vi "Write VISA Resource.vi"(8 "error in (no error)":errorcluster, 10 "VISA Resource":refnum<visa-resource-name>, 11 "Instrument.lvclass in":refnum<class "Instrument.lvclass">) -> (0 "error out":errorcluster, 3 "Instrument.lvclass out":refnum<class "Instrument.lvclass">)   [LabVIEW 2015, in "Instrument.lvclass"]
uses:
  Instrument.lvclass
  Instrument.lvclass/Instrument.ctl
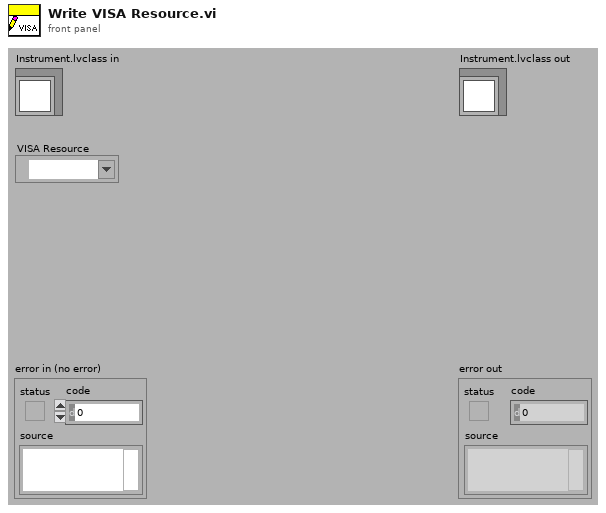
[diagram p1: front panel]
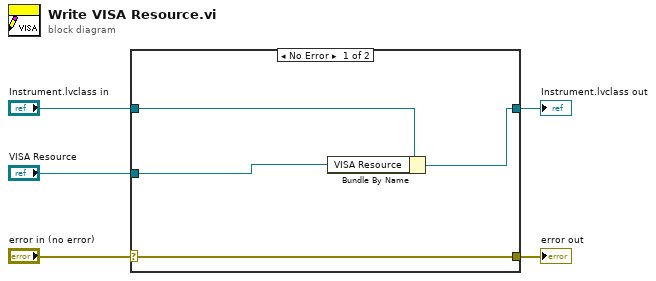
[diagram p0: block diagram]
diagram:
  n1 = case shown="No Error" "error in (no error)" {
    selector: "error in (no error)" -> [w9 w10]
    tunnel: [w9 w10] -> w4
    tunnel: [w7 w11] -> w2
    tunnel: "Instrument.lvclass in" -> [w8 w11]
    tunnel: "VISA Resource" -> [w6 _]
    frame No Error {
      n2 = Bundle By Name(cluster=w8, "VISA Resource"=w6) -> (w7:refnum<class "Instrument.lvclass">)
    }
    frame Error {
    }
  }
  "error out" <- w4
  "Instrument.lvclass out" <- w2
